vi "PH_Cont-601k_PSU.PC Flash Interval.vi"(0 "VI in":refnum<vi>, 2 "Flash Interval [s]":dbl, 5 "error in (no error)":errorcluster) -> (14 "VI out":refnum<vi>, 17 "\"Flash Interval\" changed":bool, 19 "error out":errorcluster)   [LabVIEW 2014, in "PH_Cont-601k_PSU.lvlib"]
uses:
  PH_Cont-601k_PSU.lvlib
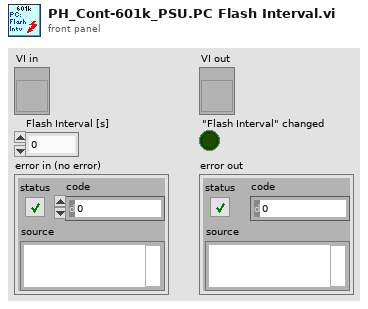
[diagram p1: front panel]
types:
  T1 = typedef "PH_Cont-601k_PSU.lvlib/PH_Cont-601k_PSU.i attribute.ctl" = cluster{"GUI Refs":T2, "Interlock":bool, "Service ID applied Voltage":i32, "Device Settings":cluster{"Configuration":T3, "Flash Interval [s]":dbl, "Mode":T4, "Voltage [V]":u16, "Charge":bool, "VISA resource name":refnum<visa-resource-name>}, "Readyness":T5, "Information":cluster{"VISA resource name":refnum<visa-resource-name>, "Tagname Power On":string, "Interlock":cluster{"Instance":string, "Tagname":string}, "Limits [V]":cluster{"Lower":dbl, "Upper":dbl}, "Tagname PSU On":string}, "R2S":bool, "Charge is allowed":bool}
  T2 = typedef "PH_Cont-601k_PSU.lvlib/PH_Cont-601k_PSU.GUI Refs.ctl" = cluster{"Power On":refnum<vi>, "Hard- and Software":refnum<vi>, "Device Status":refnum<vi>, "Device Error":refnum<vi>, "Configuration":refnum<vi>, "Flash Interval [s]":refnum<vi>, "Interlock":refnum<vi>, "Interlock Indicator":refnum<vi>, "Voltage [V]":refnum<vi>, "Readyness":refnum<vi>, "Mode":refnum<vi>, "Reset Error":refnum<vi>, "Expert working":refnum<vi>, "Charge":refnum<vi>, "PSU On":refnum<vi>}
  T3 = typedef "PH_Cont-601k_PSU.lvlib/PH_Cont-601k_PSU.Configuration.ctl" = u16
  T4 = typedef "PH_Cont-601k_PSU.lvlib/PH_Cont-601k_PSU.Mode.ctl" = enum32{"STOP", "STANDBY", "READY", "EMISSION", "ERROR"}
  T5 = typedef "PH_Cont-601k_PSU.lvlib/PH_Cont-601k_PSU.Readyness.ctl" = cluster{"Program":T6, "Device":T7}
  T6 = typedef "PH_Cont-601k_PSU.lvlib/PH_Cont-601k_PSU.Readyness Program.ctl" = enum32{"OFF", "POWER", "INTERLOCK"}
  T7 = typedef "PH_Cont-601k_PSU.lvlib/PH_Cont-601k_PSU.Readyness Device.ctl" = enum32{"OFF", "CONNECTING", "CONNECTED", "OPERATING", "EOC", "ERROR"}
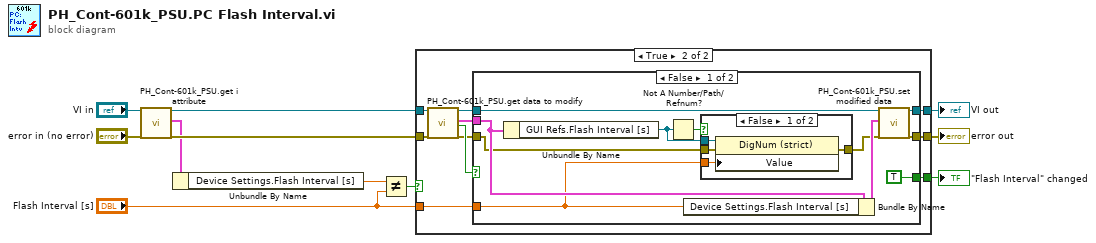
[diagram p0: block diagram]
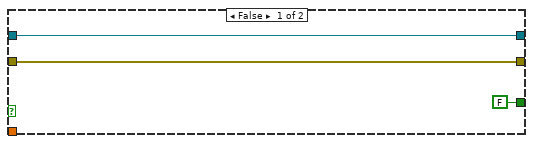
[diagram p2: hidden frame]
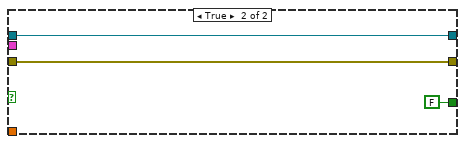
[diagram p4: hidden frame]
diagram:
  n1 = call "PH_Cont-601k_PSU.get i attribute.vi"("i ref in"="VI in", "error in (no error)"="error in (no error)") -> ("i ref out"=w8:refnum<vi>, "i attribute"=w7:T1, "error out"=w9:errorcluster)  [unwired: 15 in]
  n2 = Unbundle By Name(w7) -> ("Device Settings.Flash Interval [s]"=w6:dbl)
  n3 = Not Equal?(x=w6, y="Flash Interval [s]") -> (x != y?=w5:bool)
  n4 = case shown="True" w5 {
    tunnel: [w14 w22] -> w11
    tunnel: [w13 w19] -> w10
    tunnel: w9 -> [w13 w18]
    tunnel: w8 -> [w14 w17]
    tunnel: "Flash Interval [s]" -> [_ w16]
    tunnel: [FALSE w15] -> w1
    frame False {
    }
    frame True {
      n5 = call "PH_Cont-601k_PSU.get data to modify.vi"("i ref in"=w17, "error in (no error)"=w18) -> ("i ref out"=w21:refnum<vi>, "i attribute"=w23:T1, "timed out"=w24:bool, "error out"=w20:errorcluster)  [unwired: 14 in]
      n6 = case shown="False" w24 {
        tunnel: [w32 w42] -> w19
        tunnel: w20 -> [w28 w42]
        tunnel: w21 -> [w31 w43]
        tunnel: [w33 w43] -> w22
        tunnel: w23 -> [w30 _]
        tunnel: w16 -> [w27 _]
        tunnel: [TRUE FALSE] -> w15
        frame False {
          n7 = Unbundle By Name(w30) -> ("GUI Refs.Flash Interval [s]"=w25:refnum<vi>)
          n8 = Not A Number/Path/Refnum?(number/path/refnum=w25) -> (NaN/Path/Refnum?=w26:bool)
          n9 = Bundle By Name(cluster=w30, "Device Settings.Flash Interval [s]"=w27) -> (w35:T1)
          n10 = case shown="False" w26 {
            tunnel: [w39 w40] -> w34
            tunnel: w28 -> [w38 w40]
            tunnel: w25 -> [w37 _]
            tunnel: w27 -> [w36 _]
            frame False {
              n11 = property class="DigNum (strict)"(reference=w37, error in=w38, "Value"=w36) -> (error out=w39:errorcluster)  [unwired: 1 out]
            }
            frame True {
            }
          }
          n12 = call "PH_Cont-601k_PSU.set modified data.vi"("i ref in"=w31, "i attribute"=w35, "error in (no error)"=w34) -> ("i ref out"=w33:refnum<vi>, "error out"=w32:errorcluster)  [unwired: 15 in]
        }
        frame True {
        }
      }
    }
  }
  "VI out" <- w11
  "error out" <- w10
  "\"Flash Interval\" changed" <- w1
